vi "RT Driver VI.vi"(6 "Device Clock":string, 9 "Device Inputs FIFO":refnum<k33>, 10 "Device Outputs FIFO":refnum<k33>, 11 "Device Reference":T1 format="%.0x") -> ()   [LabVIEW 2016, in "Async UDP Engine.lvlib"]
uses:
  Async UDP Engine.lvlib
  <vilib>/NI Veristand/Custom Device API/Custom Device Item Ref.ctl
  <vilib>/NI Veristand/Custom Device API/Custom Device Channel Type.ctl
  <vilib>/NI Veristand/Custom Device API/Custom Device API.lvlib
  <vilib>/NI Veristand/Custom Device Tools/Custom Device Utility Library/Custom Device Utility Library.lvlib
panel:
  out "Timeout Error":bool
  in  "Initialization Status Notifier":refnum<notifier>
  in  "Status Notifier":refnum<notifier>
  # "Custom Device Template\nv1.0"
  # "Use this template as a starting point for creating a custom device code module. The input controls shown here are specially named controls that the system will use to provide the device loop with data. The controls are not required for the device loop to run. For instance, if the device doesn't produce any output data, then you don't need the Device Outputs FIFO control. If you do use these controls, however, they need to have these exact names to be functional."
  # "The optional status notifier element is used to notify the RT engine of the last state of the custom device, and to indicate the device has completed execution. If this control is not used, a default No Error value is returned to the system when the device finishes execution.\n\nNote: This error state is not checked until the system shuts down. Use an output status channel to send more immediate status values to the system."
  # "This optional input can be used to send the VeriStand Engine the final status of the custom device initalization process. If this control exists on the custom device front panel, the VeriStand Engine will wait for a status update before starting up. If the custom device reports an error, that will abort the execution of the current configuration in the VeriStand Engine.\n\nThis control can be deleted if the custom device does not need to send the initialization status update."
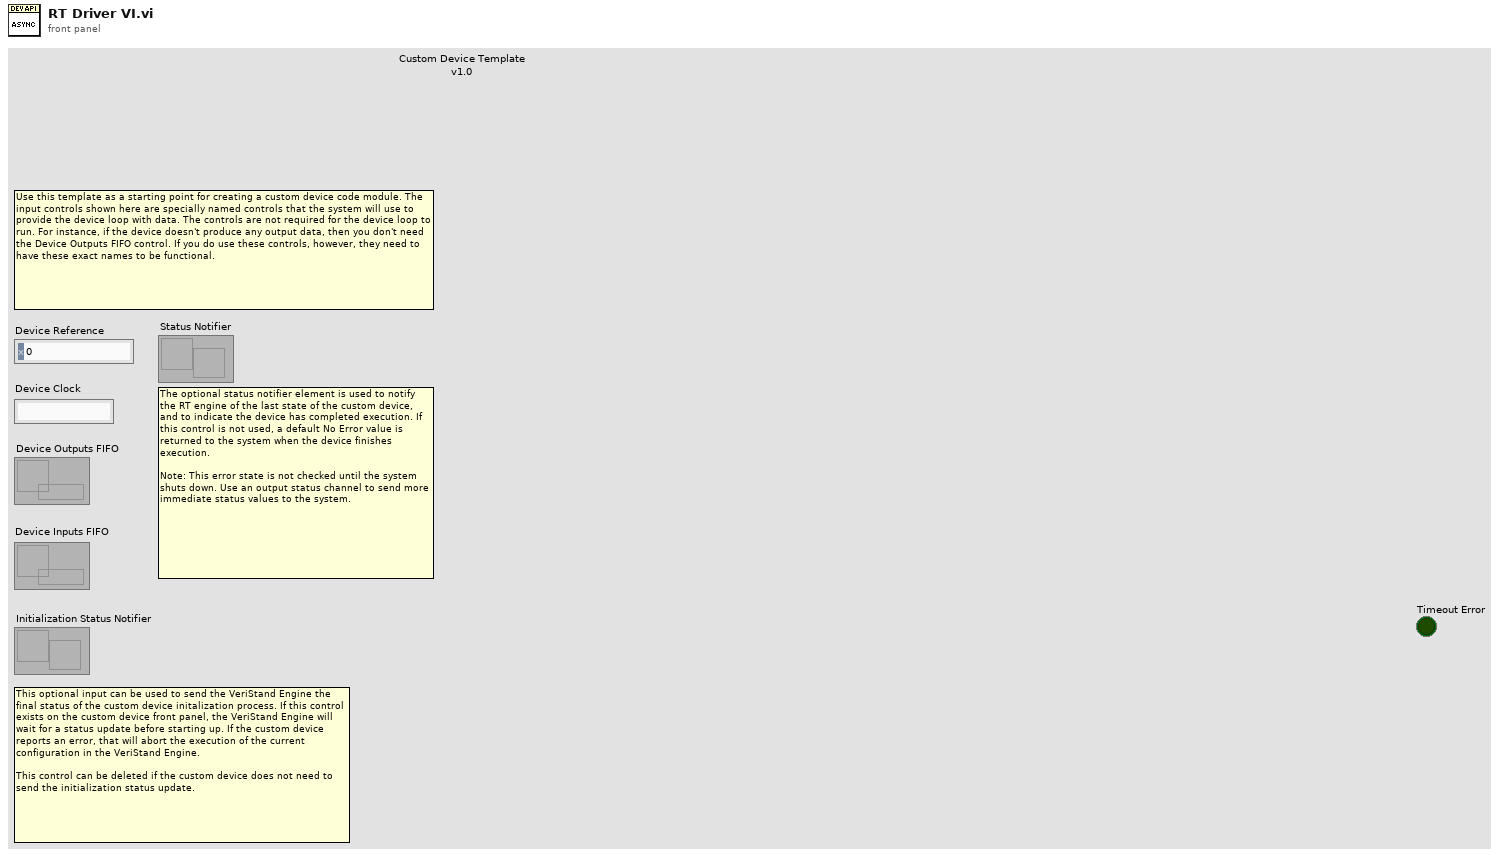
[diagram p1: front panel]
types:
  T1 = typedef "Custom Device API.lvlib/Custom Device Item Ref.ctl" = u64
  T2 = typedef "Custom Device API.lvlib/Custom Device Channel Type.ctl" = enum16{"Input", "Output"}
  T3 = typedef "Custom Device API.lvlib/Custom Device Engine Event Ref.ctl" = refnum<event-registration>
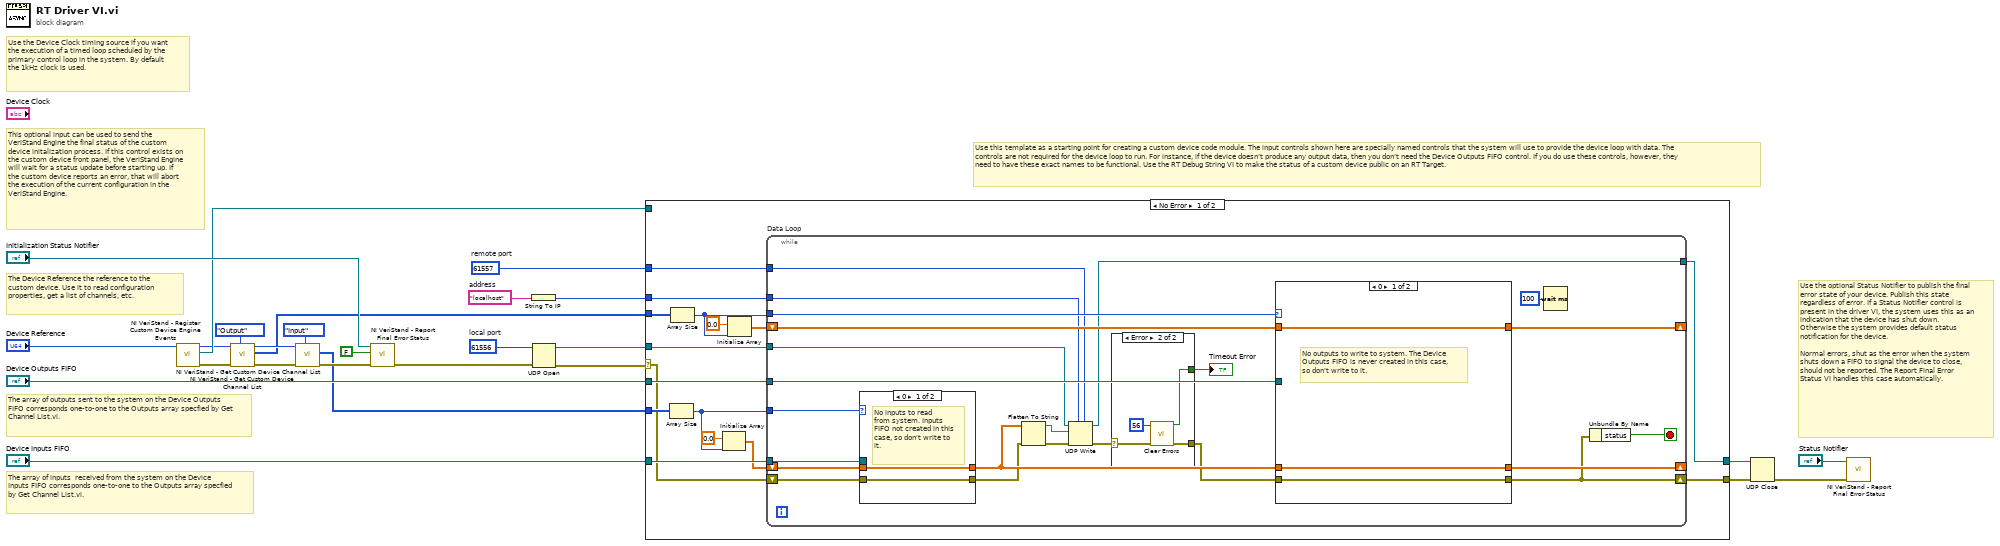
[diagram p0: block diagram]
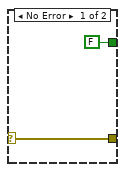
[diagram p2: hidden frame]
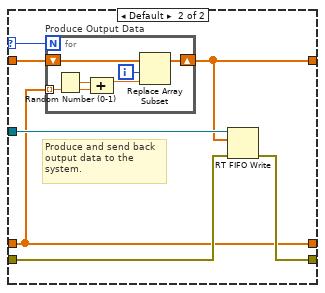
[diagram p3: hidden frame]
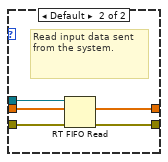
[diagram p4: hidden frame]
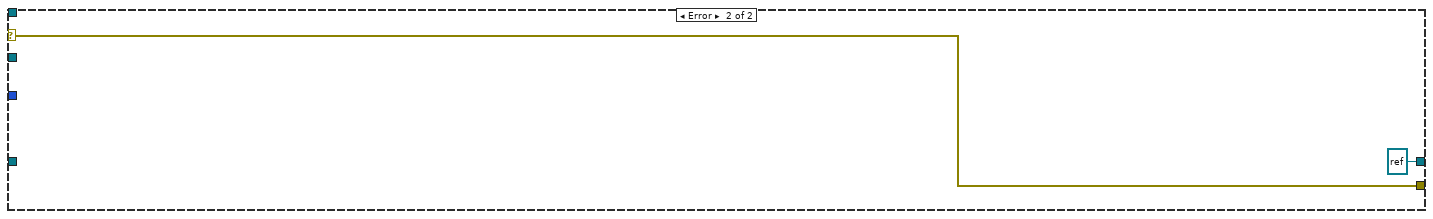
[diagram p5: hidden frame]
diagram:
  w4 = u16 61557  # remote port
  w9 = u16 61556  # local port
  w10 = "localhost"  # address
  # "This optional input can be used to send the VeriStand Engine the final status of the custom device initalization process. If this control exists on the custom device front panel, the VeriStand Engine will wait for a status update before starting up. If the custom device reports an error, that will abort the execution of the current configuration in the VeriStand Engine."
  # "The array of inputs  received from the system on the Device Inputs FIFO corresponds one-to-one to the Outputs array specfied by Get Channel List.vi."
  # "Use the optional Status Notifier to publish the final error state of your device. Publish this state regardless of error. If a Status Notifier control is present in the driver VI, the system uses this as an indication that the device has shut down. Otherwise the system provides default status notification for the device.\n\nNormal errors, shut as the error when the system shuts down a FIFO to signal the device to close, should not be reported. The Report Final Error Status VI handles this case automatically."
  # "The array of outputs sent to the system on the Device Outputs FIFO corresponds one-to-one to the Outputs array specfied by Get Channel List.vi."
  # "The Device Reference the reference to the custom device. Use it to read configuration properties, get a list of channels, etc."
  # "Use the Device Clock timing source if you want the execution of a timed loop scheduled by the primary control loop in the system. By default the 1kHz clock is used."
  # "Use this template as a starting point for creating a custom device code module. The input controls shown here are specially named controls that the system will use to provide the device loop with data. The controls are not required for the device loop to run. For instance, if the device doesn't produce any output data, then you don't need the Device Outputs FIFO control. If you do use these controls, however, they need to have these exact names to be functional. Use the RT Debug String VI to make the status of a custom device public on an RT Target."
  n1 = call <vilib>:"NI VeriStand - Register Custom Device Engine Events.vi"("Device Ref in"="Device Reference") -> ("error out"=w26:errorcluster, "Custom Device Engine Event Ref"=w14:T3, "Device Ref out"=w12:T1)  [unwired: 8 in]
  n2 = call <vilib>:"NI VeriStand - Get Custom Device Channel List.vi"("Channel Type"=Custom_Device_Channel_Type."Output", "error in (no error)"=w26, "Device Ref in"=w12) -> ("error out"=w19:errorcluster, "Specified Channel Ref List"=w16:T1[], "Device Ref out"=w20:T1)  [unwired: 6 out]
  n3 = call <vilib>:"NI VeriStand - Get Custom Device Channel List.vi"("Channel Type"=Custom_Device_Channel_Type."Input", "error in (no error)"=w19, "Device Ref in"=w20) -> ("error out"=w25:errorcluster, "Specified Channel Ref List"=w17:T1[])  [unwired: 7 out]
  n4 = call <vilib>:"NI VeriStand - Report Final Error Status.vi"("error in (no error)"=w25, "Filter FIFO & Shutdown Errors (T)"=FALSE ("Filter FIFO Errors (T)"), "Status Notifier"="Initialization Status Notifier") -> ("error out"=w8:errorcluster)  [unwired: 8 out]
  n5 = String To IP(1:w10) -> (0:w5:u32)
  n6 = UDP Open(8:w8, 11:w9) -> (port=w6:refnum<k16>, 0:w7:errorcluster)  [unwired: 3 in, 1 out]
  n7 = case shown="No Error" w7 {
    selector: w7 -> [w31 w96]
    tunnel: "Device Outputs FIFO" -> [w42 _]
    tunnel: "Device Inputs FIFO" -> [w41 _]
    tunnel: w17 -> [w35 _]
    tunnel: w16 -> [w34 _]
    tunnel: w14 -> [_ _]
    tunnel: [w32 w96] -> w3
    tunnel: w6 -> [w30 _]
    tunnel: w5 -> [w29 _]
    tunnel: w4 -> [w28 _]
    tunnel: [w27 refnum<k16> refnum ("connection ID out")] -> w1
    frame No Error {
      n8 = Array Size(array=w35) -> (size(s)=w33:i32)
      n9 = Array Size(array=w34) -> (size(s)=w36:i32)
      n10 = Initialize Array(0.0 ("element"), w33) -> (w37:dbl[])
      n11 = Initialize Array(0.0 ("element"), w36) -> (w38:dbl[])
      n12 = while "Data Loop" {
        shift-right: [w63] -> _
        shift-left: w37 -> [w64]
        shift-right: [w56] -> w32
        shift-left: w31 -> [w65]
        shift-right: [w61] -> _
        shift-left: w38 -> [w62]
        tunnel: w36 -> [w58]
        tunnel: w42 -> [w60]
        tunnel: w41 -> [w59]
        tunnel: w33 -> [w57]
        tunnel: w30 -> [w46]
        tunnel: w29 -> [w45]
        tunnel: w28 -> [w44]
        tunnel: [w43] -> w27
        stop <- w55 stop-if-true
        n13 = case shown="0" w57 {
          tunnel: w59 -> [_ w94]
          tunnel: w64 -> [w89 w93]
          tunnel: [w89 w92] -> w53
          tunnel: [w88 w91] -> w52
          tunnel: w65 -> [w88 w90]
          frame 0 {
            # "No inputs to read\nfrom system. Inputs FIFO not created in this case, so don't write to it."
          }
          frame Default {
            # "Read input data sent from the system."
            n14 = RT FIFO Read(0:w94, 1:w93, 3:w90) -> (9:w92:dbl[], 11:w91:errorcluster)  [unwired: 4 out]
          }
        }
        n15 = Flatten To String(anything=w53, error in (no error)=w52) -> (data string=w47:string, error out=w49:errorcluster)  [unwired: 2 in, 1 out]
        n16 = UDP Write(address=w45, port or service name=w44, connection ID=w46, data in=w47, 8:w49) -> (error out=w51:errorcluster, 3:w43:refnum<k16>)  [unwired: 1 in]
        n17 = case shown="Error" w51 {
          selector: w51 -> [w67 w71]
          tunnel: [w67 w69] -> w48
          tunnel: [FALSE ("specific error cleared?") w68] -> w50
          frame No Error {
          }
          frame Error {
            n18 = call <vilib>:"Clear Errors.vi"("error in (no error)"=w71, "specific error code to clear (0: all)"=56) -> ("error out"=w69:errorcluster, "specific error cleared?"=w68:bool)  [unwired: 4 in]
          }
        }
        "Timeout Error" <- w50
        n19 = case shown="0" w58 {
          selector: w58 -> [_ w75]
          tunnel: w60 -> [_ w81]
          tunnel: w62 -> [w74 w80]
          tunnel: w53 -> [w73 w76]
          tunnel: w48 -> [w72 w79]
          tunnel: [w72 w78] -> w56
          tunnel: [w74 w77] -> w61
          tunnel: [w73 w76] -> w63
          frame 0 {
            # "No outputs to write to system. The Device Outputs FIFO is never created in this case, so don't write to it."
          }
          frame Default {
            # "Produce and send back output data to the system."
            n20 = for "Produce Output Data" {
              N: w75 -> [_]
              shift-right: [w86] -> w77
              shift-left: w80 -> [w87]
              tunnel: w76 -> [w82] mode=indexing
              i -> [w85]
              n21 = Random Number (0-1)() -> (number: 0 to 1=w84:dbl)
              n22 = Compound Arithmetic op=ADD(w84, w82) -> (w83:dbl)
              n23 = Replace Array Subset(array=w87, new element=w83, index=w85) -> (w86:dbl[])
            }
            n24 = RT FIFO Write(0:w81, 1:w77, 3:w79) -> (11:w78:errorcluster)  [unwired: 1 in, 4 out]
          }
        }
        n25 = Wait (ms)(milliseconds to wait=u32 100) -> ()  [unwired: 1 out]
        n26 = Unbundle By Name(w56) -> ("status"=w55:bool)
      }
    }
    frame Error {
    }
  }
  n27 = UDP Close(connection ID=w1, 8:w3) -> (error out=w2:errorcluster)  [unwired: 1 out]
  n28 = call <vilib>:"NI VeriStand - Report Final Error Status.vi"("error in (no error)"=w2, "Status Notifier"="Status Notifier") -> ()  [unwired: 1 in, 9 out]
